vi "LeCroy_Crystallization.vi"() -> ()   [LabVIEW 2020]
doc: "This example shows how to use autosetup and acquire a waveform on a single channel for acquiring waveforms in a loop until stopped by user."
uses:
  controls/Save.ctl
  Public/Data/Read Single Sequence.vi
  <vilib>/Utility/file.llb/Write Delimited Spreadsheet (DBL).vi
  LeCroy Wave Series.lvlib
panel:
  in  "loop, ms":i32=50
  out "XY Graph":cluster{dbl[], dbl[]}(graph)
  in  "Calc":bool
  out "#points reduced":i32
  in  "Reduce factor":dbl=1.0
  out "#points":i32
  in  "Folder":path
  in  "Name":string
  in  "Save":T1
  out "error out":errorcluster
  in  "Reset?":bool
  in  "Perform Auto Setup?":bool
  in  "Timeout (10000 ms)":u32=2000
  in  "Source (0: Channel 1)":u16(ring) items=["Channel 1", "Channel 2", "Channel 3", "Channel 4", "Memory 1", "Memory 2", "Memory 3", "Memory 4", "Function 1", "Function 2", "Function 3", "Function 4", "Function 5", "Function 6", "Function 7", "Function 8"]
  in  "stop":bool
  out "Waveform Data":waveform(dbl)(graph)
  in  "VISA resource name":refnum<visa-resource-name>="VICP::129.175.100.26"
  # "(c) 2008 - 2012 NATIONAL INSTRUMENTS.  ALL RIGHTS RESERVED."
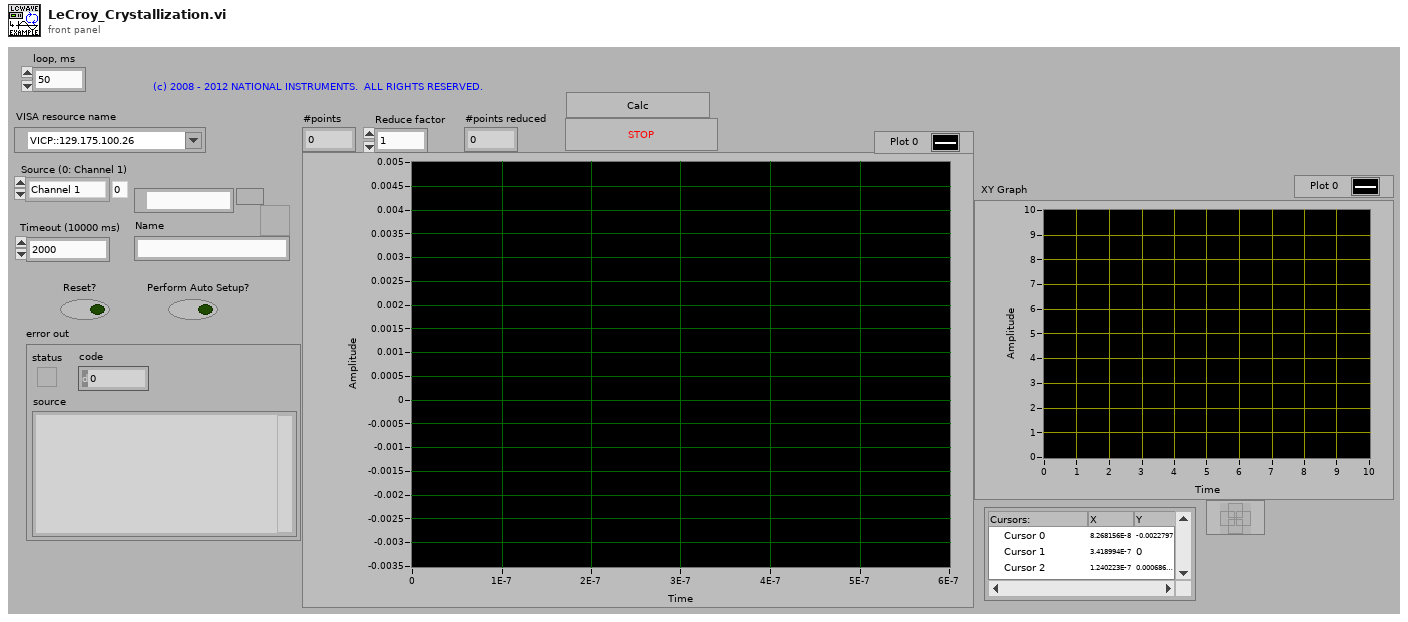
[diagram p1: front panel]
types:
  T1 = typedef "Save.ctl" = bool
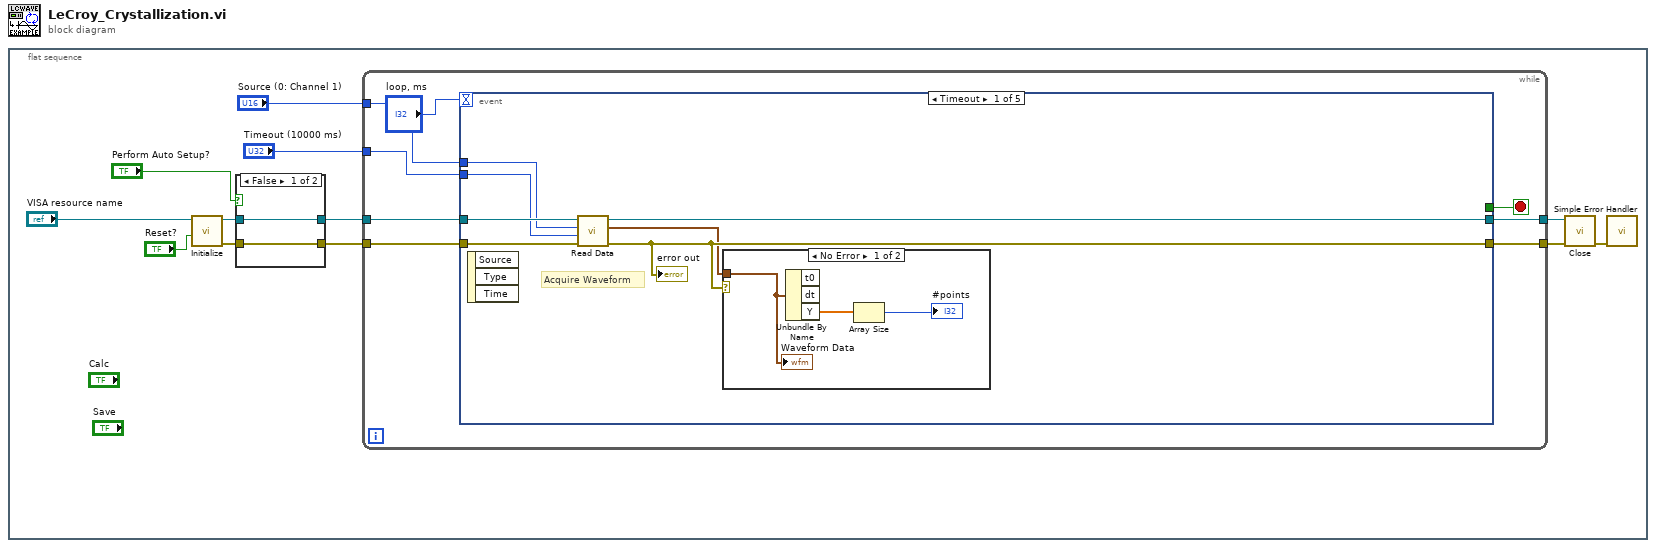
[diagram p0: block diagram]
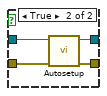
[diagram p2: hidden frame]
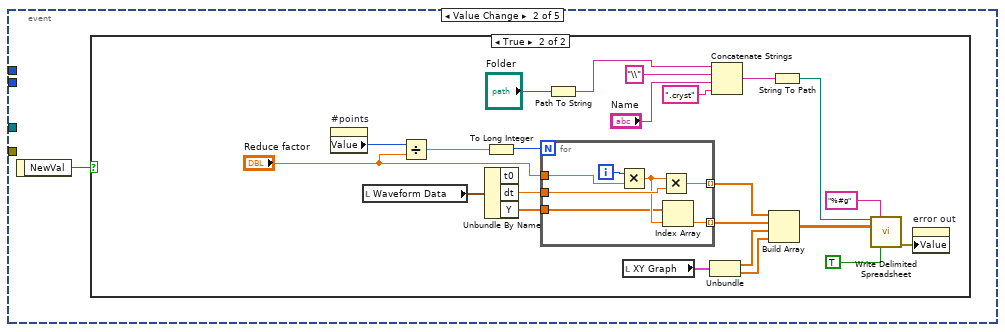
[diagram p4: hidden frame]
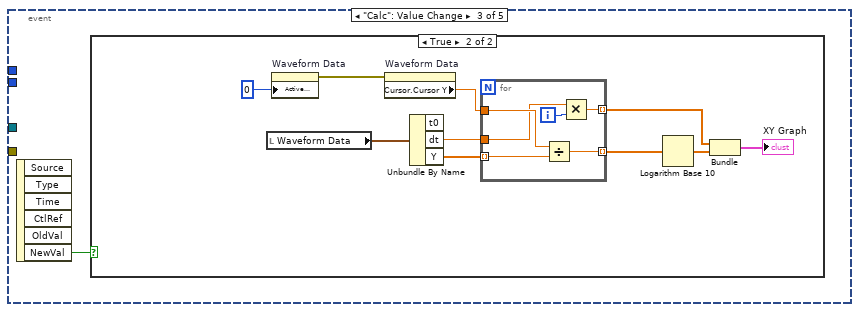
[diagram p6: hidden frame]
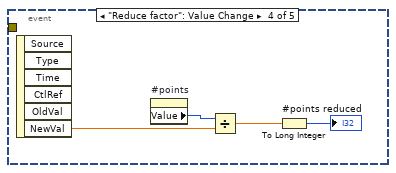
[diagram p8: hidden frame]
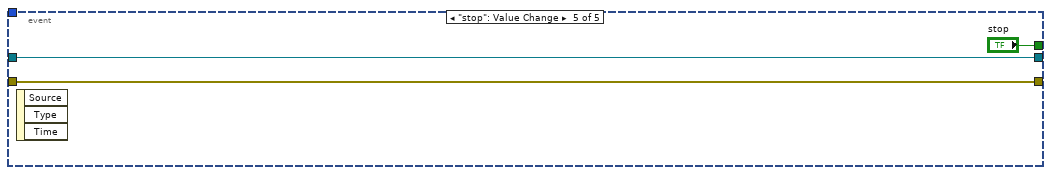
[diagram p9: hidden frame]
diagram:
  n1 = flat-sequence {
    frame #0 {
      n2 = call "Initialize.vi"("Reset? (T: Yes)"="Reset?", "VISA resource name"="VISA resource name") -> ("error out"=w9:errorcluster, "VISA resource name out"=w8:refnum<visa-resource-name>)  [unwired: 8 in]
      n3 = case shown="False" "Perform Auto Setup?" {
        tunnel: w9 -> [w13 w18]
        tunnel: w8 -> [w14 w17]
        tunnel: [w14 w16] -> w7
        tunnel: [w13 w15] -> w6
        frame False {
        }
        frame True {
          n4 = call "Autosetup.vi"("error in (no error)"=w18, "VISA resource name"=w17) -> ("error out"=w15:errorcluster, "VISA resource name out"=w16:refnum<visa-resource-name>)  [unwired: 8 in]
        }
      }
      n5 = while {
        tunnel: w7 -> [w26]
        tunnel: w6 -> [w25]
        tunnel: [w24] -> w11
        tunnel: "Source (0: Channel 1)" -> [w23]
        tunnel: "Timeout (10000 ms)" -> [w22]
        tunnel: [w19] -> w1
        stop <- w21 stop-if-true
        n6 = event shown="[0] Timeout" {
          selector: _ -> [_ _ _ _ _]
          dyn-events: _ -> [_ _ _ _ _]
          timeout: "loop, ms" -> [_ _ _ _ _]
          tunnel: w26 -> [w33 _ _ _ w90]
          tunnel: w25 -> [w32 _ _ _ w89]
          tunnel: [w31 _ _ _ w90] -> w24
          tunnel: [_ _ _ _ "stop"] -> w21
          tunnel: w23 -> [w30 _ _ _ _]
          tunnel: w22 -> [w29 _ _ _ _]
          tunnel: [w28 _ _ _ w89] -> w19
          event Timeout {
            # "Acquire Waveform"
            n7 = event-data() -> ()  [unwired: 1 in, 3 out]
            n8 = call-poly "Read Data.vi"("error in (no error)"=w32, "Timeout (10000 ms)"=w29, "Source (0: Channel 1)"=w30, "VISA resource name"=w33) -> ("error out"=w28:errorcluster, "Waveform Data"=w27:waveform(dbl), "VISA resource name out"=w31:refnum<visa-resource-name>)  [unwired: 5 in]
            "error out" <- w28
            n9 = case shown="No Error" w28 {
              tunnel: w27 -> [w36 _]
              frame No Error {
                n10 = Unbundle By Name(w36) -> ("Y"=w35:dbl[])  [unwired: 2 out]
                n11 = Array Size(array=w35) -> (size(s)=→"#points":i32)
                "Waveform Data" <- w36
              }
              frame Error {
              }
            }
          }
          event Value Change {
            n12 = event-data() -> ("NewVal"=w37:T1)  [unwired: 1 in]
            n13 = case shown="True" w37 {
              frame False {
              }
              frame True {
                n14 = property on="#points" class="DigNum (strict)"() -> ("Value"=w45:i32)  [unwired: 2 in, 2 out]
                n15 = local read "Waveform Data"() -> (w60:waveform(dbl))
                n16 = Divide(x=w45, y="Reduce factor") -> (x/y=w44:dbl)
                n17 = Unbundle By Name(w60) -> ("dt"=w59:dbl, "Y"=w57:dbl[])  [unwired: 1 out]
                n18 = To Long Integer(number=w44) -> (32bit integer=w43:i32)
                n19 = for {
                  N: w43 -> [_]
                  tunnel: w57 -> [w62]
                  tunnel: w59 -> [w67]
                  tunnel: [w66] -> w58 mode=indexing
                  tunnel: "Reduce factor" -> [w64]
                  tunnel: [w61] -> w41 mode=indexing
                  i -> [w65]
                  n20 = Multiply(x=w65, y=w64) -> (x*y=w63:dbl)
                  n21 = Multiply(x=w63, y=w67) -> (x*y=w66:dbl)
                  n22 = Index Array(array=w62, index=w63) -> (element=w61:dbl)
                }
                n23 = Path To String(path="Folder") -> (string=w47:string)
                n24 = local read "XY Graph"() -> (w40:cluster{dbl[], dbl[]})
                n25 = Unbundle(w40) -> (w39:dbl[], w38:dbl[])
                n26 = Concatenate Strings(w47, "\\" ("string"), "Name", ".cryst" ("string")) -> (w54:string)
                n27 = Build Array(w58, w41, w39, w38) -> (w52:dbl[][])
                n28 = String To Path(string=w54) -> (path=w50:path)
                n29 = call-poly <vilib>:"Write Delimited Spreadsheet.vi"("file path (dialog if empty)"=w50, "format (%.3f)"="%#g", "2D data"=w52, "transpose? (no:F)"=TRUE ("transpose? (F)")) -> ("error out"=w49:errorcluster)  [unwired: 10 in, 1 out]
                n30 = property on="error out" class="Clust (strict)"("Value"=w49) -> ()  [unwired: 2 in, 2 out]
              }
            }
          }
          event "Calc": Value Change {
            n31 = event-data() -> ("NewVal"=w68:bool)  [unwired: 1 in, 5 out]
            n32 = case shown="True" w68 {
              frame False {
              }
              frame True {
                n33 = local read "Waveform Data"() -> (w76:waveform(dbl))
                n34 = property on="Waveform Data" class="WFGraph (strict)"("Active Cursor"=u32 0) -> (error out=w77:errorcluster)  [unwired: 2 in, 1 out]
                n35 = property on="Waveform Data" class="WFGraph (strict)"(error in=w77) -> ("Cursor.Cursor Y"=w73:dbl)  [unwired: 1 in, 2 out]
                n36 = Unbundle By Name(w76) -> ("dt"=w72:dbl, "Y"=w74:dbl[])  [unwired: 1 out]
                n37 = for {
                  tunnel: [w84] -> w75 mode=indexing
                  tunnel: w74 -> [w83] mode=indexing
                  tunnel: w73 -> [w82]
                  tunnel: w72 -> [w80]
                  tunnel: [w79] -> w71 mode=indexing
                  i -> [w81]
                  n38 = Divide(x=w82, y=w83) -> (x/y=w84:dbl)
                  n39 = Multiply(x=w80, y=w81) -> (x*y=w79:dbl)
                }
                n40 = Logarithm Base 10(1:w75) -> (0:w70:dbl[])
                n41 = Bundle(w71, w70) -> (→"XY Graph":cluster{dbl[], dbl[]})  [unwired: 1 in]
              }
            }
          }
          event "Reduce factor": Value Change {
            n42 = event-data() -> ("NewVal"=w88:dbl)  [unwired: 1 in, 5 out]
            n43 = property on="#points" class="DigNum (strict)"() -> ("Value"=w87:i32)  [unwired: 2 in, 2 out]
            n44 = Divide(x=w87, y=w88) -> (x/y=w86:dbl)
            n45 = To Long Integer(number=w86) -> (32bit integer=→"#points reduced":i32)
          }
          event "stop": Value Change {
            n46 = event-data() -> ()  [unwired: 1 in, 3 out]
          }
        }
      }
      n47 = call "Close.vi"("error in (no error)"=w1, "VISA resource name"=w11) -> ("error out"=w12:errorcluster)  [unwired: 9 in]
      n48 = call <vilib>:"Simple Error Handler.vi"("error in (no error)"=w12) -> ()  [unwired: 4 in, 5 out]
    }
  }
